vi "Update Targeting Units.vi"(0 "Targeting Units":T3(array[cluster]), 1 "Scope Position":T4, 5 "Object In [pix]":T1(array[cluster]), 11 "error in (no error)":errorcluster, 12 "FOV":cluster{"X [um]":dbl, "Y [um]":dbl} {"Y [um]" format="%.2f"; "X [um]" format="%.2f"}, 13 "Image Area":cluster{"X":u32, "Y":u32}, 14 "Transformation Matrix":T2) -> (4 "Traced Objects Out [um]":T5(array[cluster]), 15 "error out":errorcluster)   [LabVIEW 2012, in "Visual Analyser.lvlib"]
uses:
  Visual Analyser.lvlib
  <vilib>/Analysis/Matrix/Datatypes/RealMatrix.ctl
  <vilib>/Analysis/Matrix/NI_Matrix.lvlib
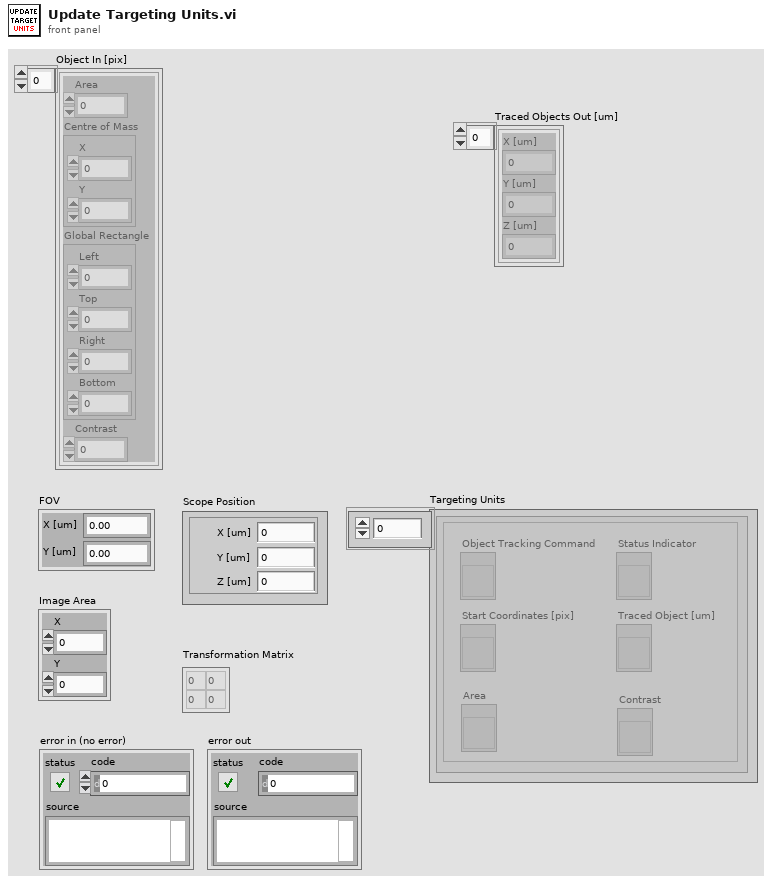
[diagram p1: front panel]
types:
  T1 = cluster{"Area":dbl, "Centre of Mass":cluster{"X":dbl, "Y":dbl}, "Global Rectangle":cluster{"Left":dbl, "Top":dbl, "Right":dbl, "Bottom":dbl}, "Contrast":dbl}[]
  T2 = typedef "NI_Matrix.lvlib/RealMatrix.ctl" = dbl[][]
  T3 = cluster{"Object Tracking Command":refnum<vi>, "Status Indicator":refnum<vi>, "Start Coordinates [pix]":refnum<vi>, "Traced Object [um]":refnum<vi>, "Area":refnum<vi>, "Contrast":refnum<vi>}[]
  T4 = cluster{"X [um]":dbl, "Y [um]":dbl, "Z [um]":dbl}
  T5 = cluster{"X [um]":dbl, "Y [um]":dbl, "Z [um]":dbl}[]
  T6 = cluster{"Area":dbl, "Centre of Mass":cluster{"X":dbl, "Y":dbl}, "Global Rectangle":cluster{"Left":dbl, "Top":dbl, "Right":dbl, "Bottom":dbl}, "Contrast":dbl}
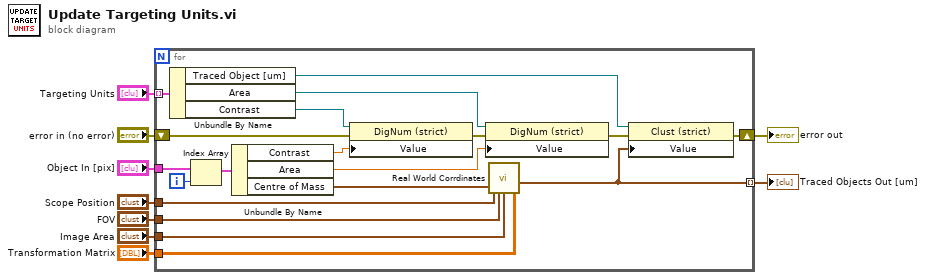
[diagram p0: block diagram]
diagram:
  n1 = for {
    tunnel: "Targeting Units" -> [w28] mode=indexing
    shift-right: [w26] -> w2
    shift-left: "error in (no error)" -> [w11]
    tunnel: "Object In [pix]" -> [w24]
    tunnel: "Scope Position" -> [w22]
    tunnel: "Image Area" -> [w21]
    tunnel: "FOV" -> [w20]
    tunnel: "Transformation Matrix" -> [w19]
    tunnel: [w18] -> w9 mode=indexing
    i -> [w23]
    n2 = Unbundle By Name(w28) -> ("Traced Object [um]"=w17:refnum<vi>, "Area"=w15:refnum<vi>, "Contrast"=w12:refnum<vi>)
    n3 = Index Array(array=w24, index=w23) -> (element=w27:T6)
    n4 = Unbundle By Name(w27) -> ("Contrast"=w10:dbl, "Area"=w14:dbl, "Centre of Mass"=w25:cluster{"X":dbl, "Y":dbl})
    n5 = property class="DigNum (strict)"(reference=w12, error in=w11, "Value"=w10) -> (error out=w13:errorcluster)  [unwired: 1 out]
    n6 = property class="DigNum (strict)"(reference=w15, error in=w13, "Value"=w14) -> (error out=w16:errorcluster)  [unwired: 1 out]
    n7 = call "Real World Corrdinates.vi"("Transformation Matrix"=w19, "coordinates [pix]"=w25, "FOV"=w20, "Scope Position"=w22, "Image Area"=w21) -> ("Target Coordinates"=w18:T4)  [unwired: 6 in]
    n8 = property class="Clust (strict)"(reference=w17, error in=w16, "Value"=w18) -> (error out=w26:errorcluster)  [unwired: 1 out]
  }
  "error out" <- w2
  "Traced Objects Out [um]" <- w9
